vi "Load ProtoFile.vi"(8 "error in (no error)":errorcluster, 10 "File Name":string, 11 "File Base path":path) -> (0 "error out":errorcluster, 3 "protoFile ref out":u64)   [LabVIEW 2019, in "gRPC Scripting Tools.lvlib"]
uses:
  gRPC Scripting Tools.lvlib
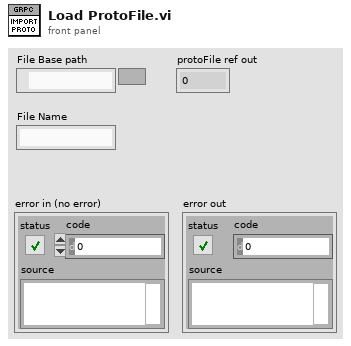
[diagram p1: front panel]
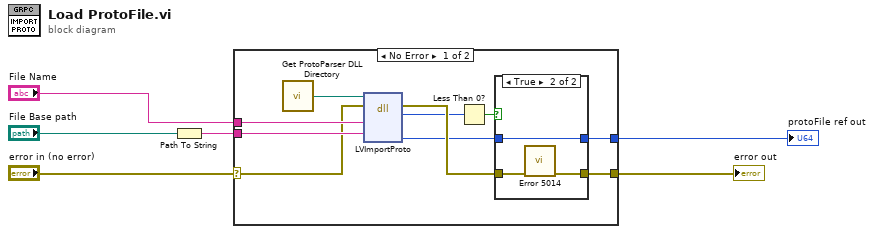
[diagram p0: block diagram]
diagram:
  n1 = Path To String(path="File Base path") -> (string=w6:string)
  n2 = case shown="No Error" "error in (no error)" {
    selector: "error in (no error)" -> [w14 w22]
    tunnel: w6 -> [w16 _]
    tunnel: "File Name" -> [w15 _]
    tunnel: [w7 _] -> w3
    tunnel: [w11 w22] -> w1
    frame No Error {
      n3 = call "Get ProtoParser DLL Directory.vi"() -> ("Proto Parser Directory"=w13:path)
      n4 = dll-call lib="C:/Users/XEnderMD/Desktop/LV gRPC/labview source/gRPC Scripting Tools/Proto Parser API/dll/labview_grpc_generator.dll" fn="LVImportProto"(path in=w13, error in=w14, "protoName"=w15, "SearchPaths"=w16) -> (error out=w12:errorcluster, "return type"=w10:i32, "protoDescription"=w8:u64)  [unwired: 4 in, 1 out]
      n5 = Less Than 0?(x=w10) -> (x < 0?=w9:bool)
      n6 = case shown="True" w9 {
        tunnel: w12 -> [w17 w21]
        tunnel: [w17 w20] -> w11
        tunnel: w8 -> [w18 w19]
        tunnel: [w18 w19] -> w7
        frame False {
        }
        frame True {
          n7 = call "Error 5014.vi"("error in (no error)"=w21) -> ("error out"=w20:errorcluster)  [unwired: 10 in]
        }
      }
    }
    frame Error {
    }
  }
  "protoFile ref out" <- w3
  "error out" <- w1
